vi "selected_columns.vi"(11 "eigen value (real)":dbl[](array[numeric])) -> (3 "Selected":bool[](array[boolean]))   [LabVIEW 2014]
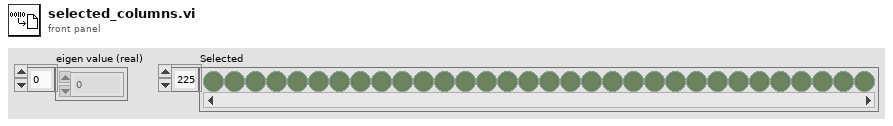
[diagram p1: front panel]
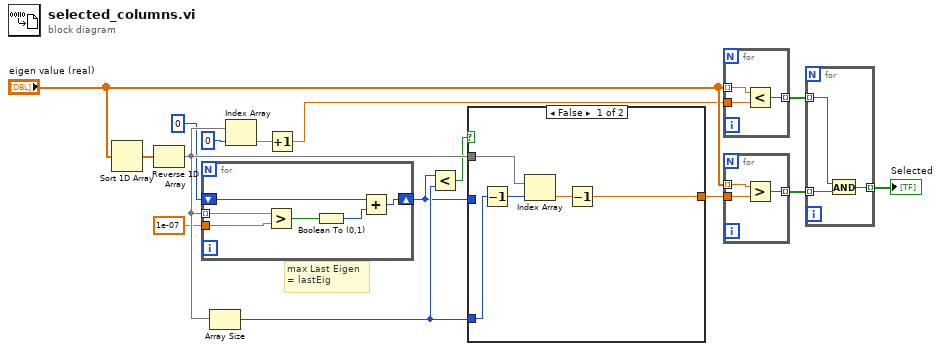
[diagram p0: block diagram]
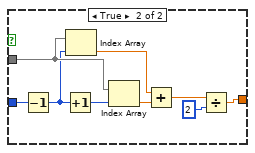
[diagram p2: hidden frame]
diagram:
  # "max Last Eigen\n= lastEig"
  n1 = Sort 1D Array(array="eigen value (real)") -> (sorted array=w1:dbl[])
  n2 = Reverse 1D Array(array=w1) -> (reversed array=w8:dbl[])
  n3 = for {
    tunnel: w8 -> [w20] mode=indexing
    tunnel: 1e-07 -> [w21]
    shift-right: [w17] -> w5
    shift-left: i16 0 -> [w16]
    n4 = Greater?(x=w20, y=w21) -> (0:w19:bool)
    n5 = Boolean To (0,1)(Boolean=w19) -> (0, 1=w18:i16)
    n6 = Add(x=w16, y=w18) -> (x+y=w17:i16)
  }
  n7 = Array Size(array=w8) -> (size(s)=w6:i32)
  n8 = Index Array(array=w8, index=0) -> (element=w10:dbl)
  n9 = Increment(x=w10) -> (x+1=w11:dbl)
  n10 = Less?(x=w5, y=w6) -> (x < y?=w4:bool)
  n11 = case shown="False" w4 {
    tunnel: w5 -> [_ w35]
    tunnel: w8 -> [w26 w34]
    tunnel: [w22 w27] -> w7
    tunnel: w6 -> [w25 _]
    frame False {
      n12 = Decrement(x=w25) -> (x-1=w24:i32)
      n13 = Index Array(array=w26, index=w24) -> (element=w23:dbl)
      n14 = Decrement(x=w23) -> (x-1=w22:dbl)
    }
    frame True {
      n15 = Decrement(x=w35) -> (x-1=w33:i16)
      n16 = Increment(x=w33) -> (x+1=w32:i16)
      n17 = Index Array(array=w34, index=w33) -> (element=w31:dbl)
      n18 = Index Array(array=w34, index=w32) -> (element=w30:dbl)
      n19 = Add(x=w31, y=w30) -> (x+y=w29:dbl)
      n20 = Divide(x=w29, y=i16 2) -> (x/y=w27:dbl)
    }
  }
  n21 = for {
    tunnel: "eigen value (real)" -> [w38] mode=indexing
    tunnel: w11 -> [w37]
    tunnel: [w36] -> w12 mode=indexing
    n22 = Less?(x=w38, y=w37) -> (x < y?=w36:bool)
  }
  n23 = for {
    tunnel: "eigen value (real)" -> [w41] mode=indexing
    tunnel: w7 -> [w40]
    tunnel: [w39] -> w13 mode=indexing
    n24 = Greater?(x=w41, y=w40) -> (0:w39:bool)
  }
  n25 = for {
    tunnel: w12 -> [w44] mode=indexing
    tunnel: w13 -> [w43] mode=indexing
    tunnel: [w42] -> w14 mode=indexing
    n26 = And(x=w44, y=w43) -> (x .and. y?=w42:bool)
  }
  "Selected" <- w14
